vi "example.vi"   [LabVIEW 2018]
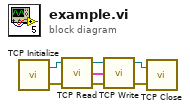
[diagram p0: block diagram]
diagram:
  n1 = call "TCP Initialize.vi"() -> ("error out"=w7:errorcluster, "connection ID"=w1:refnum<k5>)  [unwired: 2 in]
  n2 = call "TCP Read.vi"("error in (no error)"=w7, "connection ID"=w1) -> ("error out"=w6:errorcluster, "Data read"=w5:cluster{"Array of Motor Speeds":dbl[]}, "connection ID out"=w2:refnum<k5>)  [unwired: 1 in]
  n3 = call "TCP Write.vi"("error in (no error)"=w6, "Data to Write"=w5, "connection ID"=w2) -> ("error out"=w4:errorcluster, "connection ID out"=w3:refnum<k5>)  [unwired: 1 in]
  n4 = call "TCP Close.vi"("error in (no error)"=w4, "connection ID"=w3) -> ()  [unwired: 2 in]
